vi "Write Variable.vi"(8 "error in (no error)":errorcluster, 9 "Data":variant, 10 "variable":string="llab_038~d003(TEST_TABLE--voltage 3(volts))", 11 "Data.PG in":refnum<class "Data.PGSQL.lvclass">) -> (0 "error out":errorcluster, 1 "Wrote to DB?":bool, 3 "Data.PG out":refnum<class "Data.PGSQL.lvclass">)   [LabVIEW 2013, in "Data.PGSQL.lvclass"]
uses:
  Data.PGSQL.lvclass
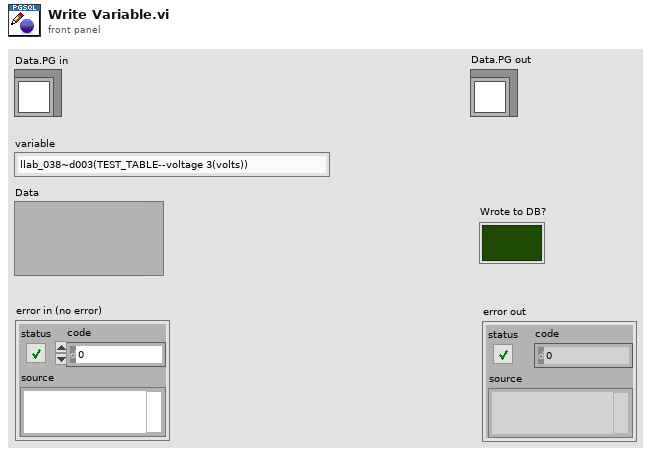
[diagram p1: front panel]
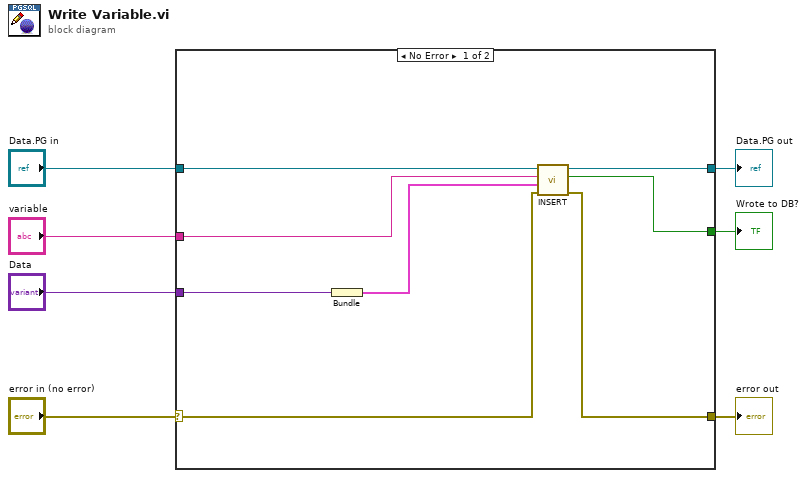
[diagram p0: block diagram]
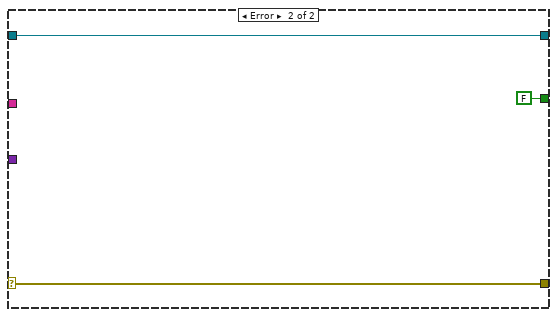
[diagram p2: hidden frame]
diagram:
  n1 = case shown="No Error" "error in (no error)" {
    selector: "error in (no error)" -> [w10 w18]
    tunnel: "Data.PG in" -> [w15 w17]
    tunnel: [w9 FALSE ("Wrote to DB?")] -> w6
    tunnel: "variable" -> [w14 _]
    tunnel: "Data" -> [w13 _]
    tunnel: [w12 w17] -> w3
    tunnel: [w8 w18] -> w1
    frame No Error {
      n2 = Bundle("Data"=w13) -> (w11:cluster{"Data":variant})  [unwired: 1 in]
      n3 = call "INSERT.vi"("error in"=w10, "Data"=w11, "Path(s)"=w14, "Data.PG in"=w15) -> ("error out"=w8:errorcluster, "Wrote to DB?"=w9:bool, "Data.PG out"=w12:refnum<class "Data.PGSQL.lvclass">)  [unwired: 5 in]
    }
    frame Error {
    }
  }
  "Wrote to DB?" <- w6
  "Data.PG out" <- w3
  "error out" <- w1
